vi "DLStatus-Com-exec.vi"(8 "error in (no error)":errorcluster, 11 "DelayLine in":refnum<class "DelayLine.lvclass">) -> (0 "error out":errorcluster, 3 "DelayLine out":refnum<class "DelayLine.lvclass">)   [LabVIEW 2019, in "DelayLine.lvclass"]
uses:
  DelayLine.lvclass
  C:/Dev/TRANCON/Classes/GeneralFunctionality/GeneralFunctionality.lvclass
  dependecies/ControlsVIs/Clusters-def/DL-Reply-to-Connect-to-Client.ctl
  dependecies/ControlsVIs/Clusters-def/SERVER-Commands.ctl
  dependecies/ControlsVIs/Clusters-def/Message types.ctl
  GeneralFunctionality/GeneralFunctionality.lvclass/GeneralFunctionality.ctl
  Message/Message.lvclass
  Control/Control-Server/Control-Server.lvclass
  GeneralFunctionality/GeneralFunctionality.lvclass
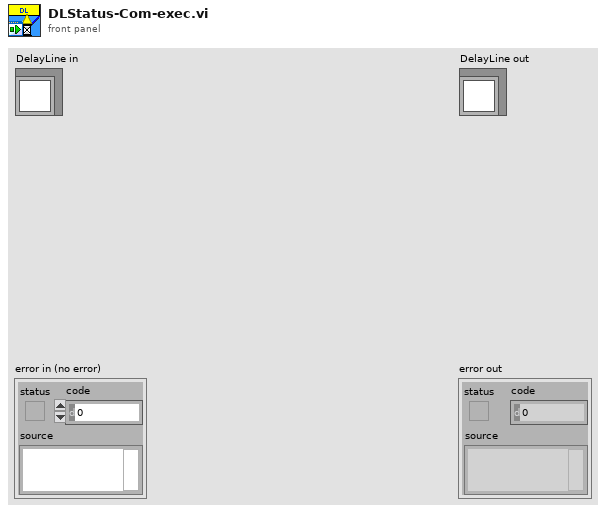
[diagram p1: front panel]
types:
  T1 = typedef "Message types.ctl" = string
  T2 = typedef "Control-Server.lvclass/SERVER-Commands.ctl" = string
  T3 = typedef "DelayLine.lvclass/DL-Reply-to-Connect-to-Client.ctl" = cluster{"on/off":bool, "pos":dbl[], "param":cluster{"min":dbl, "max":dbl, "real pos":dbl}[], "predefine_pos":dbl[][], "error":errorcluster}
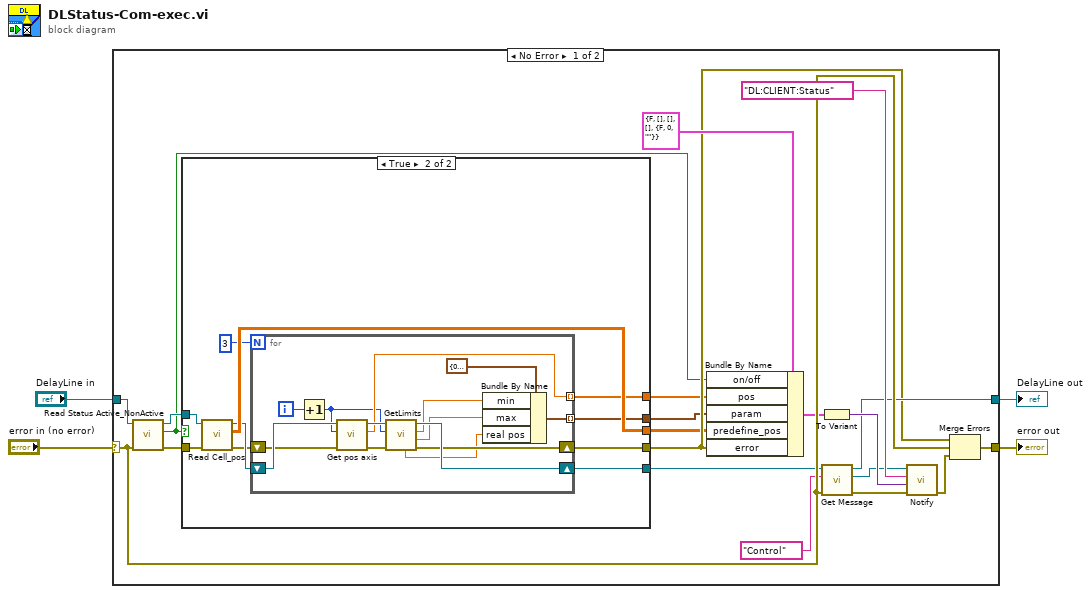
[diagram p0: block diagram]
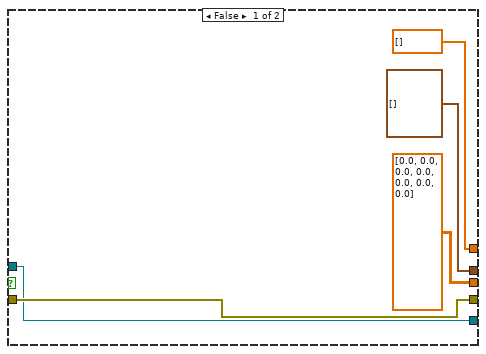
[diagram p2: hidden frame]
diagram:
  n1 = case shown="No Error" "error in (no error)" {
    selector: "error in (no error)" -> [w21 w55]
    tunnel: [w24 w55] -> w3
    tunnel: [w13 w54] -> w1
    tunnel: "DelayLine in" -> [w22 w54]
    frame No Error {
      n2 = call "Read Status Active_NonActive.vi"("error in (no error)"=w21, "GeneralFunctionality in"=w22) -> ("error out"=w10:errorcluster, "Status Active/NonActive"=w5:bool, "GeneralFunctionality out"=w11:refnum<class "DelayLine.lvclass">)  [unwired: 7 in]
      n3 = case shown="True" w5 {
        tunnel: w11 -> [w27 w38]
        tunnel: w10 -> [w29 w36]
        tunnel: [w29 w32] -> w12
        tunnel: [dbl[][] [[0.0, 0.0, 0.0, 0.0, 0.0, 0.0, 0.0]] ("Cell_pos") w39] -> w7
        tunnel: [w27 w33] -> w6
        tunnel: [dbl[] [] w31] -> w9
        tunnel: [cluster{"min":dbl, "max":dbl, "real pos":dbl}[] [] w30] -> w8
        frame False {
        }
        frame True {
          n4 = call "Read Cell_pos.vi"("error in (no error)"=w36, "DelayLine in"=w38) -> ("error out"=w34:errorcluster, "Cell_pos"=w39:dbl[][], "DelayLine out"=w35:refnum<class "DelayLine.lvclass">)  [unwired: 7 in]
          n5 = for {
            N: 3 -> [_]
            shift-right: [w50] -> w33
            shift-left: w35 -> [w49]
            shift-right: [w47] -> w32
            shift-left: w34 -> [w48]
            tunnel: [w46] -> w31 mode=indexing
            tunnel: [w41] -> w30 mode=indexing
            i -> [w53]
            n6 = Increment(x=w53) -> (x+1=w40:i32)
            n7 = call-dynamic "Get pos axis.vi"("error in (no error)"=w48, "Axis"=w40, "DelayLine in"=w49) -> ("error out"=w52:errorcluster, "Pos"=w46:dbl, "DelayLine out"=w51:refnum<class "DelayLine.lvclass">)  [unwired: 6 in]
            n8 = call-dynamic "GetLimits.vi"("error in (no error)"=w52, "Axis"=w40, "DelayLine in"=w51) -> ("error out"=w47:errorcluster, "max"=w43:dbl, "min"=w44:dbl, "DelayLine out"=w50:refnum<class "DelayLine.lvclass">, "real pos, mm"=w42:dbl)  [unwired: 4 in]
            n9 = Bundle By Name(cluster=cluster{"min":dbl, "max":dbl, "real pos":dbl} {"min"=0.0, "max"=0.0, "real pos"=0.0} ("axis"), "min"=w44, "max"=w43, "real pos"=w42) -> (w41:cluster{"min":dbl, "max":dbl, "real pos":dbl})
          }
        }
      }
      n10 = Bundle By Name(cluster=T3 {"on/off"=FALSE, "pos"=[], "param"=[], "predefine_pos"=[], "error"={"status"=FALSE, "code"=0, "source"=""}} ("output cluster"), "on/off"=w5, "pos"=w9, "param"=w8, "predefine_pos"=w7, "error"=w12) -> (w18:T3)
      n11 = To Variant(anything=w18) -> (Variant=w17:variant)
      n12 = call "Get Message.vi"("error in (no error)"=w21, "Message type"=T1 "Control", "GeneralFunctionality en entrée"=w6) -> ("error out"=w20:errorcluster, "Message.lvclass"=w15:refnum<class "Message.lvclass">, "GeneralFunctionality en sortie"=w13:refnum<class "DelayLine.lvclass">)  [unwired: 6 in]
      n13 = call "Notify.vi"("error in (no error)"=w20, "Data"=w17, "command"=T2 "DL:CLIENT:Status" ("Commands"), "Message en entrée"=w15) -> ("error out"=w19:errorcluster)  [unwired: 6 in, 1 out]
      n14 = Merge Errors(w12, w21, w19) -> (w24:errorcluster)
    }
    frame Error {
    }
  }
  "error out" <- w3
  "DelayLine out" <- w1
